vi "Read.vi"(8 "error in (no error)":errorcluster, 11 "I32 in":refnum<class "I32.lvclass">) -> (0 "error out":errorcluster, 2 "I32":i32, 3 "I32 out":refnum<class "I32.lvclass">)   [LabVIEW 2020, in "Data.lvlib" / "I32.lvclass"]
doc: "Read I32."
uses:
  I32.lvclass
  I32.lvclass/I32.ctl
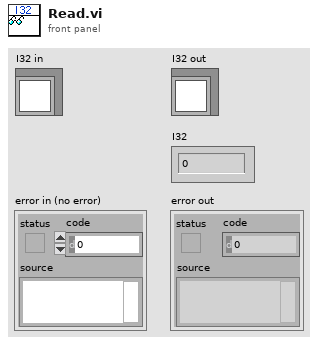
[diagram p1: front panel]
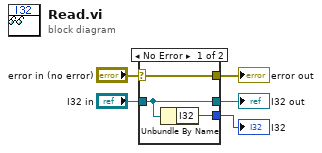
[diagram p0: block diagram]
diagram:
  n1 = case shown="No Error" "error in (no error)" {
    selector: "error in (no error)" -> [w8 w9]
    tunnel: [w8 w9] -> w4
    tunnel: [w7 w10] -> w2
    tunnel: "I32 in" -> [w7 w10]
    tunnel: [w6 _] -> w1
    frame No Error {
      n2 = Unbundle By Name(w7) -> ("I32"=w6:i32)
    }
    frame Error {
    }
  }
  "error out" <- w4
  "I32 out" <- w2
  "I32" <- w1
